vi "Xscale fudge.vi"(0 "x array":sgl[](array[numeric]), 1 "intensity array in":sgl[][](array[numeric])) -> (2 "xscale maximum":sgl, 3 "xscale minimum":sgl, 4 "intensity array out":dbl[][](array[numeric]))   [LabVIEW 2014]
panel:
  out "int array":dbl[](array[numeric])
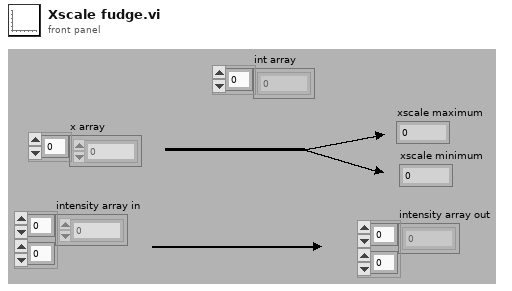
[diagram p1: front panel]
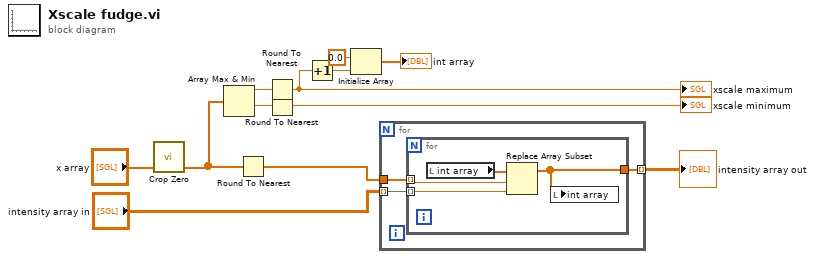
[diagram p0: block diagram]
diagram:
  n1 = call "Crop Zero.vi"("Search data"="x array") -> ("Searched data out"=w8:dbl[])  [unwired: 3 in, 1 out]
  n2 = Array Max & Min(array=w8) -> (max value=w7:dbl, min value=w6:dbl)  [unwired: 2 out]
  n3 = Round To Nearest(number=w8) -> (nearest integer value=w12:dbl[])
  n4 = Round To Nearest(number=w7) -> (nearest integer value=w4:dbl)
  "xscale maximum" <- w4
  n5 = Round To Nearest(number=w6) -> (nearest integer value=→"xscale minimum":dbl)
  n6 = Increment(x=w4) -> (x+1=w2:dbl)
  n7 = Initialize Array(0.0 ("element"), w2) -> (→"int array":dbl[])
  n8 = for {
    tunnel: w12 -> [w15]
    tunnel: "intensity array in" -> [w14] mode=indexing
    tunnel: [w13] -> w10 mode=indexing
    n9 = for {
      tunnel: w15 -> [w19] mode=indexing
      tunnel: w14 -> [w18] mode=indexing
      tunnel: [w16] -> w13
      n10 = local read "int array"() -> (w17:dbl[])
      n11 = Replace Array Subset(array=w17, new element=w18, index=w19) -> (w16:dbl[])
      n12 = local write "int array"(w16) -> ()
    }
  }
  "intensity array out" <- w10
